vi "Launch Action - NI XNET CAN Signal Logger - Executor.vi"(8 "error in (no error)":errorcluster, 11 "Executor Command":refnum<user-event>) -> (0 "error out":errorcluster)   [LabVIEW 2021, in "XNET-CAN-Signal-Logger.lvlib"]
uses:
  XNET-CAN-Signal-Logger.lvlib
  Typedef/Def-Executor Command.ctl
  NI XNET CAN Signal Logger - Executor.vi
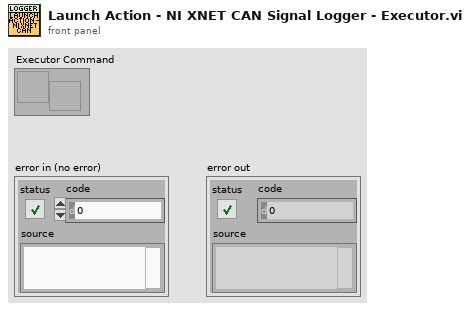
[diagram p1: front panel]
types:
  T1 = enum32{"Bad", "Idle", "Run top level", "Running"}
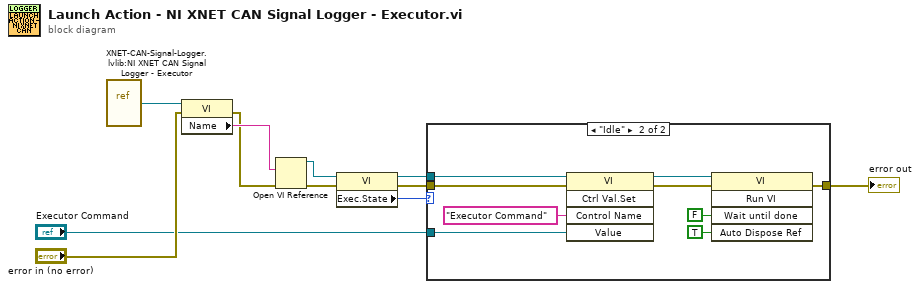
[diagram p0: block diagram]
diagram:
  n1 = vi-ref "XNET-CAN-Signal-Logger.lvlib:NI XNET CAN Signal Logger - Executor.vi"() -> (w11:refnum<vi>)
  n2 = property class="VI"(reference=w11, error in="error in (no error)") -> (error out=w9:errorcluster, "Name"=w10:string)  [unwired: 1 out]
  n3 = Open VI Reference(vi path=w10, error in (no error)=w9) -> (vi reference=w8:refnum<vi>, error out=w6:errorcluster)  [unwired: 4 in]
  n4 = property class="VI"(reference=w8, error in=w6) -> (reference out=w5:refnum<vi>, error out=w4:errorcluster, "Exec.State"=w3:T1)
  n5 = case shown="\"Idle\"" w3 {
    tunnel: "Executor Command" -> [_ w18]
    tunnel: [w12 w13] -> w7
    tunnel: w5 -> [_ w15]
    tunnel: w4 -> [w12 w14]
    frame Default {
    }
    frame "Idle" {
      n6 = invoke class="VI" method="Ctrl Val.Set"(reference=w15, error in=w14, "Control Name"="Executor Command", "Value"=w18) -> (reference out=w17:refnum<vi>, error out=w16:errorcluster)  [unwired: 1 in, 3 out]
      n7 = invoke class="VI" method="Run VI"(reference=w17, error in=w16, "Wait until done"=FALSE ("Wait Until Done"), "Auto Dispose Ref"=TRUE ("Auto Dispose Reference")) -> (error out=w13:errorcluster)  [unwired: 1 in, 4 out]
    }
  }
  "error out" <- w7
